vi "Example_guider_2.vi"() -> ()   [LabVIEW 2018]
panel:
  out "Reponse":string
  in  "B":dbl
  in  "A":dbl
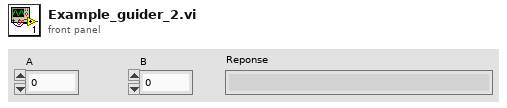
[diagram p1: front panel]
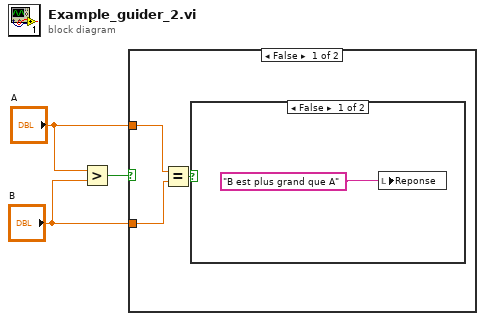
[diagram p0: block diagram]
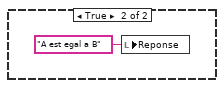
[diagram p2: hidden frame]
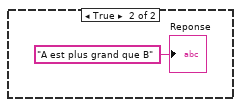
[diagram p3: hidden frame]
diagram:
  n1 = Greater?(x="A", y="B") -> (0:w3:bool)
  n2 = case shown="False" w3 {
    tunnel: "A" -> [w4 _]
    tunnel: "B" -> [w5 _]
    frame False {
      n3 = Equal?(x=w4, y=w5) -> (x = y?=w6:bool)
      n4 = case shown="False" w6 {
        frame False {
          n5 = local write "Reponse"("B est plus grand que A" ("Reponse")) -> ()
        }
        frame True {
          n6 = local write "Reponse"("A est egal a B" ("Reponse")) -> ()
        }
      }
    }
    frame True {
      "Reponse" <- "A est plus grand que B" ("Reponse")
    }
  }
